vi "数字双相码.vi"() -> ()   [LabVIEW 2013]
panel:
  in  "停止":bool
  out "波形图表":dbl[](graph)
  out "数字双相码":i8[](array[numeric])
  in  "原消息代码":u32[](array[numeric])
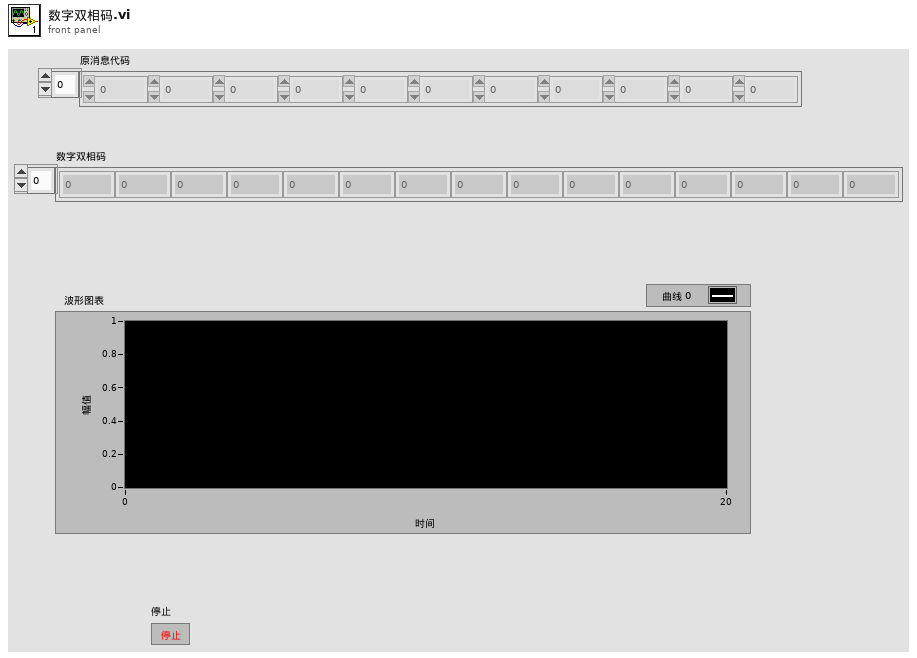
[diagram p1: front panel]
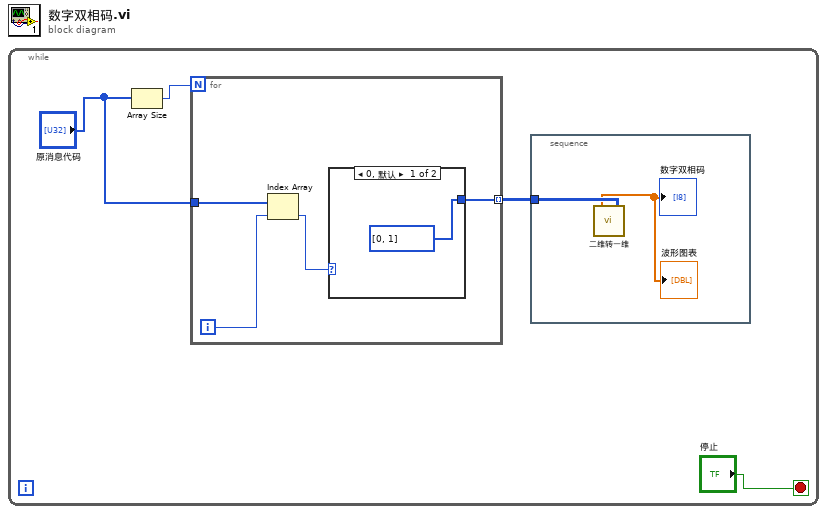
[diagram p0: block diagram]
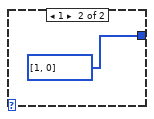
[diagram p2: hidden frame]
diagram:
  n1 = while {
    stop <- "停止" stop-if-true
    n2 = Array Size(array="原消息代码") -> (size(s)=w4:i32)
    n3 = for {
      N: w4 -> [_]
      tunnel: "原消息代码" -> [w10]
      tunnel: [w8] -> w2 mode=indexing
      i -> [w9]
      n4 = Index Array(array=w10, index=w9) -> (element=w7:u32)
      n5 = case shown="0, 默认" w7 {
        tunnel: [i32[] [0, 1] i32[] [1, 0]] -> w8
        frame 0, Default {
        }
        frame 1 {
        }
      }
    }
    n6 = stacked-sequence {
      tunnel: w2 -> [w6]
      frame #0 {
        n7 = call "二维转一维.vi"("输入2维"=w6) -> ("输出一维"=→"数字双相码" →"波形图表":dbl[])
      }
    }
  }
